vi "GenerateAnalogWaveformPiezoTraj - Copy.vi"(8 "error in (no error)":errorcluster, 11 "SetupInfo_IN":T1={"ConfigParameters_Analog"={"JAI camera fps"=240.0, "Bi-Lateral Galvo xy scan range (V)"=0.7, "Bi-Lateral Galvo xy scan frequency (Hz)"=500, "AOM Blind percent (%)"=0.1, "AOM start blind percent (%) "=70.0, "ROI threshold"=1.0, "AO Sampling rate"=1000000.0}, "ConfigParameters_Digital"={"Steps per volume"=25.0, "Time per volume (s)"=0.4, "OG start layer"=15.0, "Objective Lin Rising Vel (micron/ms）"=1.0, "Image depth (micron)"=200.0, "OG latency (s)"=10.0, "OG repitation"=3.0, "OG end layer"=17.0, "Shock1 duration (s)"=0.001, "Shock2 duration (s)"=0.001, "Shock3 duration (s)"=0.01, "Shock4 duration (s)"=0.01, "Shock5 duration (s)"=0.1, "Shock duration_New"=[]}, "ConfigParameters_Other1"={"Frontal Galvo xy scan range (V)"=0.14, "Frontal Galvo xy scan frequency (Hz)"=500, "PFI 0 digital clock frequency"=500000.0, "Window size for layer index"=0.5, "sCMOS fps"=95.0}, "ConfigParameters_Others2"={"#Trials baseline"=6, "#Trials test"=6, "Time before acq. (s)"=360.0, "Time before test (s)"=600.0, "#Blocks acquisition"=5, "Inter-trial interval baseline (s)"=60.0, "#Trials per acquition block"=6, "Inter-block interval acquisition (s)"=360.0, "Inter-trial interval acquisition (s)"=20.0, "Flash latency (s)"=10.0, "Flash duration (s)"=3.2, "Response duration (s)"=10.0, "MaxTimeEventDetection (s)"=6, "StimType"=enum."Flash", "#MaxEvents"=6}, "ProcessParametersOut"={"stand Z vol Acquisition time (s)"=0.2631578947368421, "stand Z vol Backward time (s)"=0.13684210526315793, "Objective scan volt"=5.0, "Bi-lateral Galvo Z scan volt"=0.45, "Frontal Galvo Z scan volt"=0.37, "Objective step length (micron)"=8.0, "OG Z volet Linear Dec time (s)"=0.024, "OG Z vol Stim. steps time (s)"=0.031578947368421054, "OG Z vol Linear Acc time (s)"=0.112, "#Vol. of flash"=8, "#Vol. of shock"=1, "#Vol. bef flash"=25, "#Vol. aft flash"=17, "OG Z vol Linear Dec time (s)"=0.112, "OG Z vol time (s)"=0.39073684210526316, "Stack duration"=[0.001, 0.001, 0.01, 0.01, 0.1], "AOM stand. value size"=400000, "Plane indexing length"=0, "#Vol. blank"=0, "#Vol. blank before acq"=0, "#Vol. blank before test"=0, " #Inter-block interval acquisition (Ed-St Vol)"=0}, "WaveformParameters"={"stand Z vol Acquisition samp info"={"Fs"=1000000.0, "#s"=263158.0}, "stand Z vol Backward samp info"={"Fs"=1000000.0, "#s"=136842.0}, "OG Z vol Linear Acc samp info"={"Fs"=1000000.0, "#s"=112000.0}, "OG Z vol Stim. steps samp info"={"Fs"=1000000.0, "#s"=31579.0}, "OG Z volet Linear Dec samp info"={"Fs"=1000000.0, "#s"=24000.0}, "OG Z vol Linear Dec samp info"={"Fs"=1000000.0, "#s"=112000.0}, "OG Z vol samp info"={"Fs"=1000000.0, "#s"=390737.0}, "stand Z vol backforth samp info"={"Fs"=1000000.0, "#s"=400000.0}}, "AnalogWaveform"={"Bi-lateral Galvo Z stand waveform"={"t0"=timestamp(0 s since 1904-01-01), "dt"=1.0, "Y"=[]}, "Frontal Galvo Z stand waveform"={"t0"=timestamp(0 s since 1904-01-01), "dt"=1.0, "Y"=[]}, "Bi-lateral Galvo XY stand waveform"={"t0"=timestamp(0 s since 1904-01-01), "dt"=1.0, "Y"=[]}, "Frontal Galvo XY stand waveform"={"t0"=timestamp(0 s since 1904-01-01), "dt"=1.0, "Y"=[]}, "sCMOS stand waveform"={"t0"=timestamp(0 s since 1904-01-01), "dt"=1.0, "Y"=[]}, "Detection objective stand waveform"={"t0"=timestamp(0 s since 1904-01-01), "dt"=1.0, "Y"=[]}, "AOM stand waveform"={"t0"=timestamp(0 s since 1904-01-01), "dt"=1.0, "Y"=[]}, "PFI 0 clock stand waveform"={"t0"=timestamp(0 s since 1904-01-01), "dt"=1.0, "Y"=[]}, "Bi-lateral Galvo Z OG waveform"={"t0"=timestamp(0 s since 1904-01-01), "dt"=1.0, "Y"=[]}, "Bi-lateral Galvo XY OG waveform"={"t0"=timestamp(0 s since 1904-01-01), "dt"=1.0, "Y"=[]}, "Frontal Galvo Z OG waveform"={"t0"=timestamp(0 s since 1904-01-01), "dt"=1.0, "Y"=[]}, "Frontal Galvo XY OG waveform"={"t0"=timestamp(0 s since 1904-01-01), "dt"=1.0, "Y"=[]}, "sCMOS OG waveform"={"t0"=timestamp(0 s since 1904-01-01), "dt"=1.0, "Y"=[]}, "Detection objective OG waveform"={"t0"=timestamp(0 s since 1904-01-01), "dt"=1.0, "Y"=[]}, "AOM OG waveform"={"t0"=timestamp(0 s since 1904-01-01), "dt"=1.0, "Y"=[]}, "PFI 0 clock OG wavee"={"t0"=timestamp(0 s since 1904-01-01), "dt"=1.0, "Y"=[]}, "sCMOS blank waveform"={"t0"=timestamp(0 s since 1904-01-01), "dt"=1.0, "Y"=[]}, "All analog OG wave"=[], "All analog stand wave"=[], "All analog blank wave"=[], "BufferWaveform_Analog"=[], "Bi-lateral Galvo Z XY"={"t0"=timestamp(0 s since 1904-01-01), "dt"=1.0, "Y"=[]}, "Frontal Galvo Z XY"={"t0"=timestamp(0 s since 1904-01-01), "dt"=1.0, "Y"=[]}, "sCMOS Trigger XY"={"t0"=timestamp(0 s since 1904-01-01), "dt"=1.0, "Y"=[]}, "Detection objective XY"={"t0"=timestamp(0 s since 1904-01-01), "dt"=1.0, "Y"=[]}, "AOM XY"={"t0"=timestamp(0 s since 1904-01-01), "dt"=1.0, "Y"=[]}, "Analog_XY"=[]}, "DigitalWaveform"={"AllDigitalStandWave"=[], "AllDigialEvokedWave"=[], "AllDigialOGWave"=[], "AllDigitalPairWave_1"=[], "AllDigitalPairWave_2"=[], "AllDigitalPairWave_3"=[], "AllDigitalPairWave_4"=[], "AllDigitalPairWave_5"=[], "Plane Indexing"={"t0"=timestamp(0 s since 1904-01-01), "dt"=0.0, "Y"={"transitions"=[], "data"=[]}, "error"={"status"=FALSE, "code"=37421928, "source"=""}}, "Plane indexing P0.5 OG"={"t0"=timestamp(0 s since 1904-01-01), "dt"=0.0, "Y"={"transitions"=[], "data"=[]}, "error"={"status"=FALSE, "code"=37421928, "source"=""}}, "AllDigitalPairWaves"=[], "BufferWaveform_Digital"=[], "AllDigitalBlankWave"=[], "Digial_XY"=[], "Digital_XY_flash"=[]}, "PhysicalResource"={"PhysicalChannels_AI"="", "PhysicalChannels_AO"="", "PhysicalChannels_DO"="", "Task_AnalogOutput"="", "Task_DigitalOutput"="", "Task_AnalogInput"=""}, "ControlsRef"={"Mode_1"=refnum, "EventDetectionMode"=refnum, "Mode_2A"=refnum, "StimulationMode"=refnum, "Mode_2B"=refnum, "ErrorMeg"=refnum}} {"ConfigParameters_Other1"."Frontal Galvo xy scan frequency (Hz)" min=500 max=500; "ConfigParameters_Other1"."Frontal Galvo xy scan range (V)" min=0.0 max=1.5; "ConfigParameters_Analog"."AOM start blind percent (%)" min=10.0 max=90.0; "ConfigParameters_Analog"."AOM Blind percent (%)" min=0.1 max=100.0; "ConfigParameters_Analog"."Bi-Lateral Galvo xy scan frequency (Hz)" min=500 max=500; "ConfigParameters_Analog"."Bi-Lateral Galvo xy scan range (V)" min=0.0 max=1.5}) -> (0 "error out":errorcluster, 3 "SetupInfo_OUT":T1={"ConfigParameters_Analog"={"JAI camera fps"=240.0, "Bi-Lateral Galvo xy scan range (V)"=0.7, "Bi-Lateral Galvo xy scan frequency (Hz)"=500, "AOM Blind percent (%)"=0.1, "AOM start blind percent (%) "=70.0, "ROI threshold"=1.0, "AO Sampling rate"=1000000.0}, "ConfigParameters_Digital"={"Steps per volume"=25.0, "Time per volume (s)"=0.4, "OG start layer"=15.0, "Objective Lin Rising Vel (micron/ms）"=1.0, "Image depth (micron)"=200.0, "OG latency (s)"=10.0, "OG repitation"=3.0, "OG end layer"=17.0, "Shock1 duration (s)"=0.001, "Shock2 duration (s)"=0.001, "Shock3 duration (s)"=0.01, "Shock4 duration (s)"=0.01, "Shock5 duration (s)"=0.1, "Shock duration_New"=[]}, "ConfigParameters_Other1"={"Frontal Galvo xy scan range (V)"=0.14, "Frontal Galvo xy scan frequency (Hz)"=500, "PFI 0 digital clock frequency"=500000.0, "Window size for layer index"=0.5, "sCMOS fps"=95.0}, "ConfigParameters_Others2"={"#Trials baseline"=6, "#Trials test"=6, "Time before acq. (s)"=360.0, "Time before test (s)"=600.0, "#Blocks acquisition"=5, "Inter-trial interval baseline (s)"=60.0, "#Trials per acquition block"=6, "Inter-block interval acquisition (s)"=360.0, "Inter-trial interval acquisition (s)"=20.0, "Flash latency (s)"=10.0, "Flash duration (s)"=3.2, "Response duration (s)"=10.0, "MaxTimeEventDetection (s)"=6, "StimType"=enum."Flash", "#MaxEvents"=6}, "ProcessParametersOut"={"stand Z vol Acquisition time (s)"=0.2631578947368421, "stand Z vol Backward time (s)"=0.13684210526315793, "Objective scan volt"=5.0, "Bi-lateral Galvo Z scan volt"=0.1800000180000018, "Frontal Galvo Z scan volt"=0.14940000509752818, "Objective step length (micron)"=8.0, "OG Z volet Linear Dec time (s)"=0.024, "OG Z vol Stim. steps time (s)"=0.031578947368421054, "OG Z vol Linear Acc time (s)"=0.112, "#Vol. of flash"=8, "#Vol. of shock"=1, "#Vol. bef flash"=25, "#Vol. aft flash"=17, "OG Z vol Linear Dec time (s)"=0.112, "OG Z vol time (s)"=0.39073684210526316, "Stack duration"=[0.001, 0.001, 0.01, 0.01, 0.1], "AOM stand. value size"=400000, "Plane indexing length"=0, "#Vol. blank"=0, "#Vol. blank before acq"=0, "#Vol. blank before test"=0, " #Inter-block interval acquisition (Ed-St Vol)"=0}, "WaveformParameters"={"stand Z vol Acquisition samp info"={"Fs"=1000000.0, "#s"=263158.0}, "stand Z vol Backward samp info"={"Fs"=1000000.0, "#s"=136842.0}, "OG Z vol Linear Acc samp info"={"Fs"=1000000.0, "#s"=112000.0}, "OG Z vol Stim. steps samp info"={"Fs"=1000000.0, "#s"=31579.0}, "OG Z volet Linear Dec samp info"={"Fs"=1000000.0, "#s"=24000.0}, "OG Z vol Linear Dec samp info"={"Fs"=1000000.0, "#s"=112000.0}, "OG Z vol samp info"={"Fs"=1000000.0, "#s"=390737.0}, "stand Z vol backforth samp info"={"Fs"=1000000.0, "#s"=400000.0}}, "AnalogWaveform"={"Bi-lateral Galvo Z stand waveform"={"t0"=timestamp(0 s since 1904-01-01), "dt"=1.0, "Y"=[]}, "Frontal Galvo Z stand waveform"={"t0"=timestamp(0 s since 1904-01-01), "dt"=1.0, "Y"=[]}, "Bi-lateral Galvo XY stand waveform"={"t0"=timestamp(0 s since 1904-01-01), "dt"=1.0, "Y"=[]}, "Frontal Galvo XY stand waveform"={"t0"=timestamp(0 s since 1904-01-01), "dt"=1.0, "Y"=[]}, "sCMOS stand waveform"={"t0"=timestamp(0 s since 1904-01-01), "dt"=1.0, "Y"=[]}, "Detection objective stand waveform"={"t0"=timestamp(0 s since 1904-01-01), "dt"=1.0, "Y"=[]}, "AOM stand waveform"={"t0"=timestamp(0 s since 1904-01-01), "dt"=1.0, "Y"=[]}, "PFI 0 clock stand waveform"={"t0"=timestamp(0 s since 1904-01-01), "dt"=1.0, "Y"=[]}, "Bi-lateral Galvo Z OG waveform"={"t0"=timestamp(0 s since 1904-01-01), "dt"=1.0, "Y"=[]}, "Bi-lateral Galvo XY OG waveform"={"t0"=timestamp(0 s since 1904-01-01), "dt"=1.0, "Y"=[]}, "Frontal Galvo Z OG waveform"={"t0"=timestamp(0 s since 1904-01-01), "dt"=1.0, "Y"=[]}, "Frontal Galvo XY OG waveform"={"t0"=timestamp(0 s since 1904-01-01), "dt"=1.0, "Y"=[]}, "sCMOS OG waveform"={"t0"=timestamp(0 s since 1904-01-01), "dt"=1.0, "Y"=[]}, "Detection objective OG waveform"={"t0"=timestamp(0 s since 1904-01-01), "dt"=1.0, "Y"=[]}, "AOM OG waveform"={"t0"=timestamp(0 s since 1904-01-01), "dt"=1.0, "Y"=[]}, "PFI 0 clock OG wavee"={"t0"=timestamp(0 s since 1904-01-01), "dt"=1.0, "Y"=[]}, "sCMOS blank waveform"={"t0"=timestamp(0 s since 1904-01-01), "dt"=1.0, "Y"=[]}, "All analog OG wave"=[], "All analog stand wave"=[], "All analog blank wave"=[], "BufferWaveform_Analog"=[], "Bi-lateral Galvo Z XY"={"t0"=timestamp(0 s since 1904-01-01), "dt"=1.0, "Y"=[]}, "Frontal Galvo Z XY"={"t0"=timestamp(0 s since 1904-01-01), "dt"=1.0, "Y"=[]}, "sCMOS Trigger XY"={"t0"=timestamp(0 s since 1904-01-01), "dt"=1.0, "Y"=[]}, "Detection objective XY"={"t0"=timestamp(0 s since 1904-01-01), "dt"=1.0, "Y"=[]}, "AOM XY"={"t0"=timestamp(0 s since 1904-01-01), "dt"=1.0, "Y"=[]}, "Analog_XY"=[]}, "DigitalWaveform"={"AllDigitalStandWave"=[], "AllDigialEvokedWave"=[], "AllDigialOGWave"=[], "AllDigitalPairWave_1"=[], "AllDigitalPairWave_2"=[], "AllDigitalPairWave_3"=[], "AllDigitalPairWave_4"=[], "AllDigitalPairWave_5"=[], "Plane Indexing"={"t0"=timestamp(0 s since 1904-01-01), "dt"=0.0, "Y"={"transitions"=[], "data"=[]}, "error"={"status"=FALSE, "code"=37421928, "source"=""}}, "Plane indexing P0.5 OG"={"t0"=timestamp(0 s since 1904-01-01), "dt"=0.0, "Y"={"transitions"=[], "data"=[]}, "error"={"status"=FALSE, "code"=37421928, "source"=""}}, "AllDigitalPairWaves"=[], "BufferWaveform_Digital"=[], "AllDigitalBlankWave"=[], "Digial_XY"=[], "Digital_XY_flash"=[]}, "PhysicalResource"={"PhysicalChannels_AI"="", "PhysicalChannels_AO"="", "PhysicalChannels_DO"="", "Task_AnalogOutput"="", "Task_DigitalOutput"="", "Task_AnalogInput"=""}, "ControlsRef"={"Mode_1"=refnum, "EventDetectionMode"=refnum, "Mode_2A"=refnum, "StimulationMode"=refnum, "Mode_2B"=refnum, "ErrorMeg"=refnum}} {"ConfigParameters_Other1"."Frontal Galvo xy scan frequency (Hz)" min=500 max=500; "ConfigParameters_Other1"."Frontal Galvo xy scan range (V)" min=0.0 max=1.5; "ConfigParameters_Analog"."AOM start blind percent (%)" min=10.0 max=90.0; "ConfigParameters_Analog"."AOM Blind percent (%)" min=0.1 max=100.0; "ConfigParameters_Analog"."Bi-Lateral Galvo xy scan frequency (Hz)" min=500 max=500; "ConfigParameters_Analog"."Bi-Lateral Galvo xy scan range (V)" min=0.0 max=1.5})   [LabVIEW 2018]
uses:
  SetupInfo.ctl
  ConfigParameters_Analog.ctl
  ConfigParameters_Digital.ctl
  ConfigParameters_Others1.ctl
  ConfigParameters_Others2.ctl
  ProcessParametersOut.ctl
  WaveformParameters.ctl
  AnalogWaveform.ctl
  DigitalWaveform.ctl
  PhysicalResource.ctl
  ControlsRef.ctl
  <vilib>/Waveform/WDTOps.llb/WDT Append Waveforms DBL.vi
  <vilib>/measure/NI_MABase.lvlib
panel:
  in  "FileSamplingRate":dbl=1000.0
  in  "PiezoTrajectoryPath":path=path "D:/APP/LightSheetController_Ver8 obl/VISource/Waveform/Piezo_feedback_20201106.txt"
  out "AOM stand. value size":i32=400000
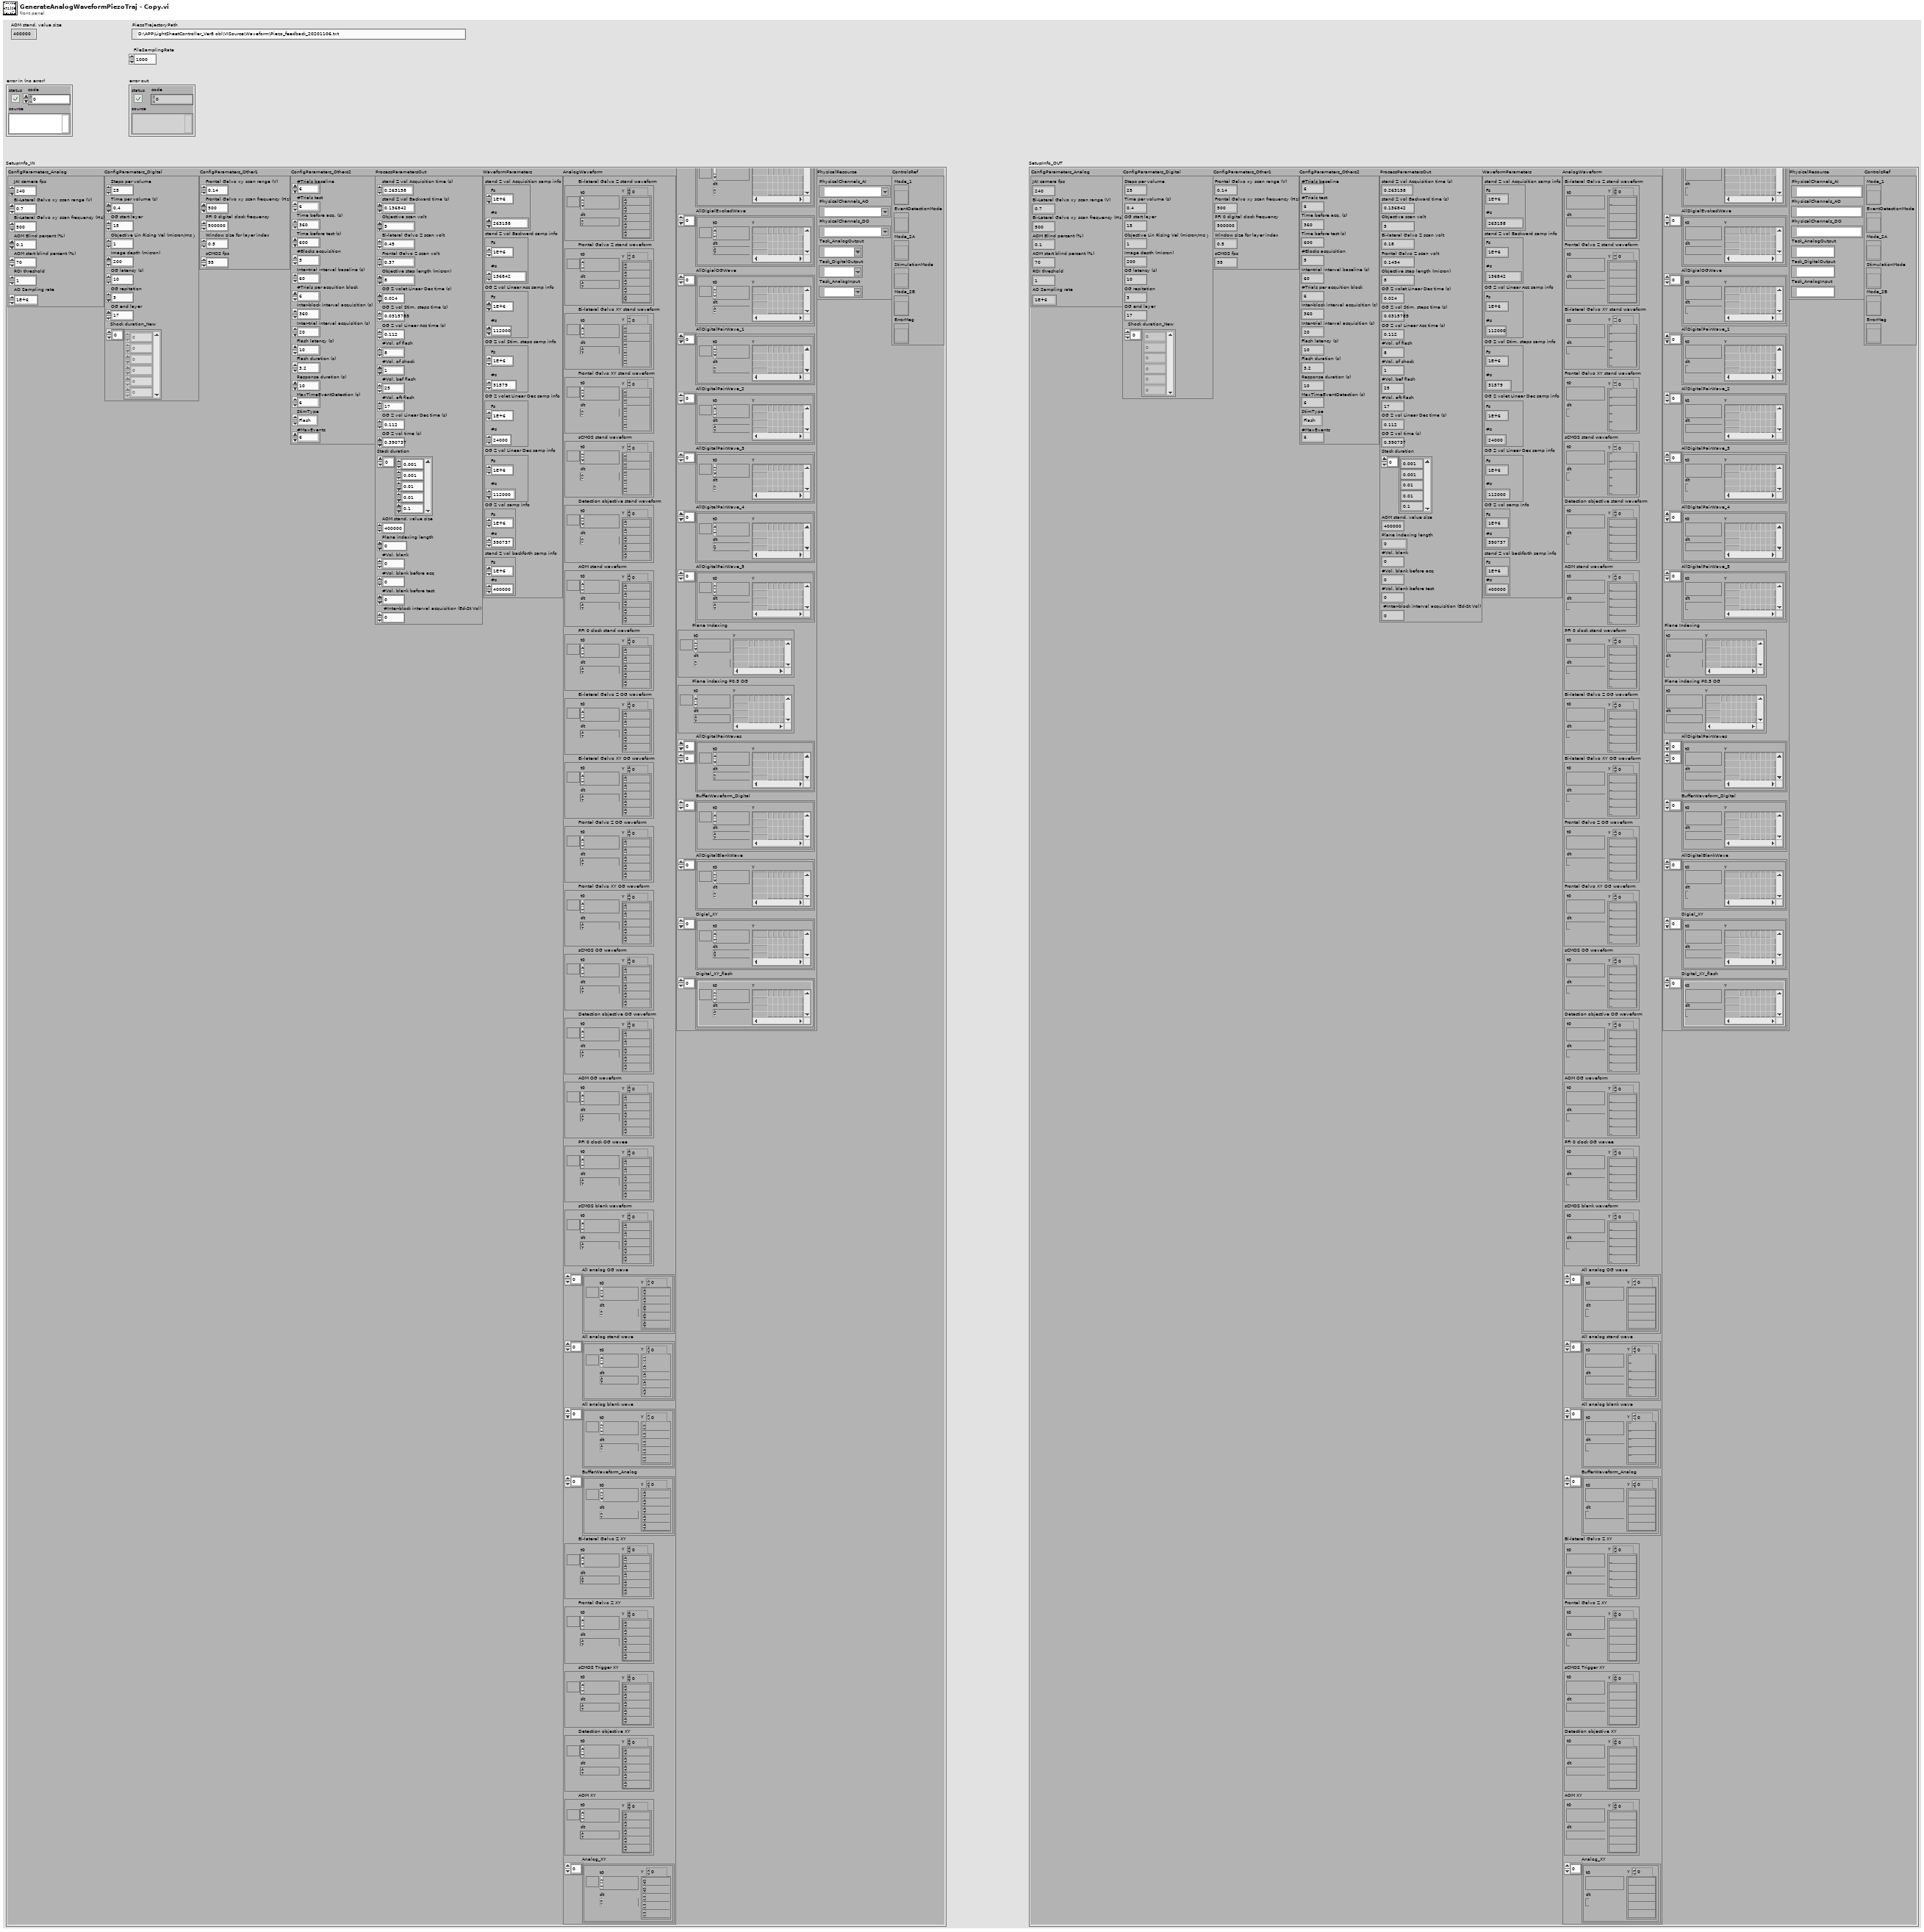
[diagram p1: front panel]
types:
  T1 = typedef "SetupInfo.ctl" = cluster{"ConfigParameters_Analog":T2, "ConfigParameters_Digital":T3, "ConfigParameters_Other1":T4, "ConfigParameters_Others2":T5, "ProcessParametersOut":T6, "WaveformParameters":T7, "AnalogWaveform":T8, "DigitalWaveform":T9, "PhysicalResource":T10, "ControlsRef":T11}
  T2 = typedef "ConfigParameters_Analog.ctl" = cluster{"JAI camera fps":dbl, "Bi-Lateral Galvo xy scan range (V)":dbl, "Bi-Lateral Galvo xy scan frequency (Hz)":i16, "AOM Blind percent (%)":dbl, "AOM start blind percent (%) ":dbl, "ROI threshold":dbl, "AO Sampling rate":dbl}
  T3 = typedef "ConfigParameters_Digital.ctl" = cluster{"Steps per volume":dbl, "Time per volume (s)":dbl, "OG start layer":dbl, "Objective Lin Rising Vel (micron/ms）":dbl, "Image depth (micron)":dbl, "OG latency (s)":dbl, "OG repitation":dbl, "OG end layer":dbl, "Shock1 duration (s)":dbl, "Shock2 duration (s)":dbl, "Shock3 duration (s)":dbl, "Shock4 duration (s)":dbl, "Shock5 duration (s)":dbl, "Shock duration_New":dbl[]}
  T4 = typedef "ConfigParameters_Others1.ctl" = cluster{"Frontal Galvo xy scan range (V)":dbl, "Frontal Galvo xy scan frequency (Hz)":i16, "PFI 0 digital clock frequency":dbl, "Window size for layer index":dbl, "sCMOS fps":dbl}
  T5 = typedef "ConfigParameters_Others2.ctl" = cluster{"#Trials baseline":i32, "#Trials test":i32, "Time before acq. (s)":dbl, "Time before test (s)":dbl, "#Blocks acquisition":i32, "Inter-trial interval baseline (s)":dbl, "#Trials per acquition block":i32, "Inter-block interval acquisition (s)":dbl, "Inter-trial interval acquisition (s)":dbl, "Flash latency (s)":dbl, "Flash duration (s)":dbl, "Response duration (s)":dbl, "MaxTimeEventDetection (s)":i32, "StimType":enum16{"Flash", "OG"}, "#MaxEvents":i32}
  T6 = typedef "ProcessParametersOut.ctl" = cluster{"stand Z vol Acquisition time (s)":dbl, "stand Z vol Backward time (s)":dbl, "Objective scan volt":dbl, "Bi-lateral Galvo Z scan volt":dbl, "Frontal Galvo Z scan volt":dbl, "Objective step length (micron)":dbl, "OG Z volet Linear Dec time (s)":dbl, "OG Z vol Stim. steps time (s)":dbl, "OG Z vol Linear Acc time (s)":dbl, "#Vol. of flash":i32, "#Vol. of shock":i32, "#Vol. bef flash":i32, "#Vol. aft flash":i32, "OG Z vol Linear Dec time (s)":dbl, "OG Z vol time (s)":dbl, "Stack duration":dbl[], "AOM stand. value size":i32, "Plane indexing length":i32, "#Vol. blank":i32, "#Vol. blank before acq":i32, "#Vol. blank before test":i32, " #Inter-block interval acquisition (Ed-St Vol)":i32}
  T7 = typedef "WaveformParameters.ctl" = cluster{"stand Z vol Acquisition samp info":cluster{"Fs":dbl, "#s":dbl}, "stand Z vol Backward samp info":cluster{"Fs":dbl, "#s":dbl}, "OG Z vol Linear Acc samp info":cluster{"Fs":dbl, "#s":dbl}, "OG Z vol Stim. steps samp info":cluster{"Fs":dbl, "#s":dbl}, "OG Z volet Linear Dec samp info":cluster{"Fs":dbl, "#s":dbl}, "OG Z vol Linear Dec samp info":cluster{"Fs":dbl, "#s":dbl}, "OG Z vol samp info":cluster{"Fs":dbl, "#s":dbl}, "stand Z vol backforth samp info":cluster{"Fs":dbl, "#s":dbl}}
  T8 = typedef "AnalogWaveform.ctl" = cluster{"Bi-lateral Galvo Z stand waveform":waveform(dbl), "Frontal Galvo Z stand waveform":waveform(dbl), "Bi-lateral Galvo XY stand waveform":waveform(dbl), "Frontal Galvo XY stand waveform":waveform(dbl), "sCMOS stand waveform":waveform(dbl), "Detection objective stand waveform":waveform(dbl), "AOM stand waveform":waveform(dbl), "PFI 0 clock stand waveform":waveform(dbl), "Bi-lateral Galvo Z OG waveform":waveform(dbl), "Bi-lateral Galvo XY OG waveform":waveform(dbl), "Frontal Galvo Z OG waveform":waveform(dbl), "Frontal Galvo XY OG waveform":waveform(dbl), "sCMOS OG waveform":waveform(dbl), "Detection objective OG waveform":waveform(dbl), "AOM OG waveform":waveform(dbl), "PFI 0 clock OG wavee":waveform(dbl), "sCMOS blank waveform":waveform(dbl), "All analog OG wave":waveform(dbl)[], "All analog stand wave":waveform(dbl)[], "All analog blank wave":waveform(dbl)[], "BufferWaveform_Analog":waveform(dbl)[], "Bi-lateral Galvo Z XY":waveform(dbl), "Frontal Galvo Z XY":waveform(dbl), "sCMOS Trigger XY":waveform(dbl), "Detection objective XY":waveform(dbl), "AOM XY":waveform(dbl), "Analog_XY":waveform(dbl)[]}
  T9 = typedef "DigitalWaveform.ctl" = cluster{"AllDigitalStandWave":digitalwaveform[], "AllDigialEvokedWave":digitalwaveform[], "AllDigialOGWave":digitalwaveform[], "AllDigitalPairWave_1":digitalwaveform[], "AllDigitalPairWave_2":digitalwaveform[], "AllDigitalPairWave_3":digitalwaveform[], "AllDigitalPairWave_4":digitalwaveform[], "AllDigitalPairWave_5":digitalwaveform[], "Plane Indexing":digitalwaveform, "Plane indexing P0.5 OG":digitalwaveform, "AllDigitalPairWaves":digitalwaveform[][], "BufferWaveform_Digital":digitalwaveform[], "AllDigitalBlankWave":digitalwaveform[], "Digial_XY":digitalwaveform[], "Digital_XY_flash":digitalwaveform[]}
  T10 = typedef "PhysicalResource.ctl" = cluster{"PhysicalChannels_AI":tag, "PhysicalChannels_AO":tag, "PhysicalChannels_DO":tag, "Task_AnalogOutput":refnum<k21>, "Task_DigitalOutput":refnum<k21>, "Task_AnalogInput":refnum<k21>}
  T11 = typedef "ControlsRef.ctl" = cluster{"Mode_1":refnum<vi>, "EventDetectionMode":refnum<vi>, "Mode_2A":refnum<vi>, "StimulationMode":refnum<vi>, "Mode_2B":refnum<vi>, "ErrorMeg":refnum<vi>}
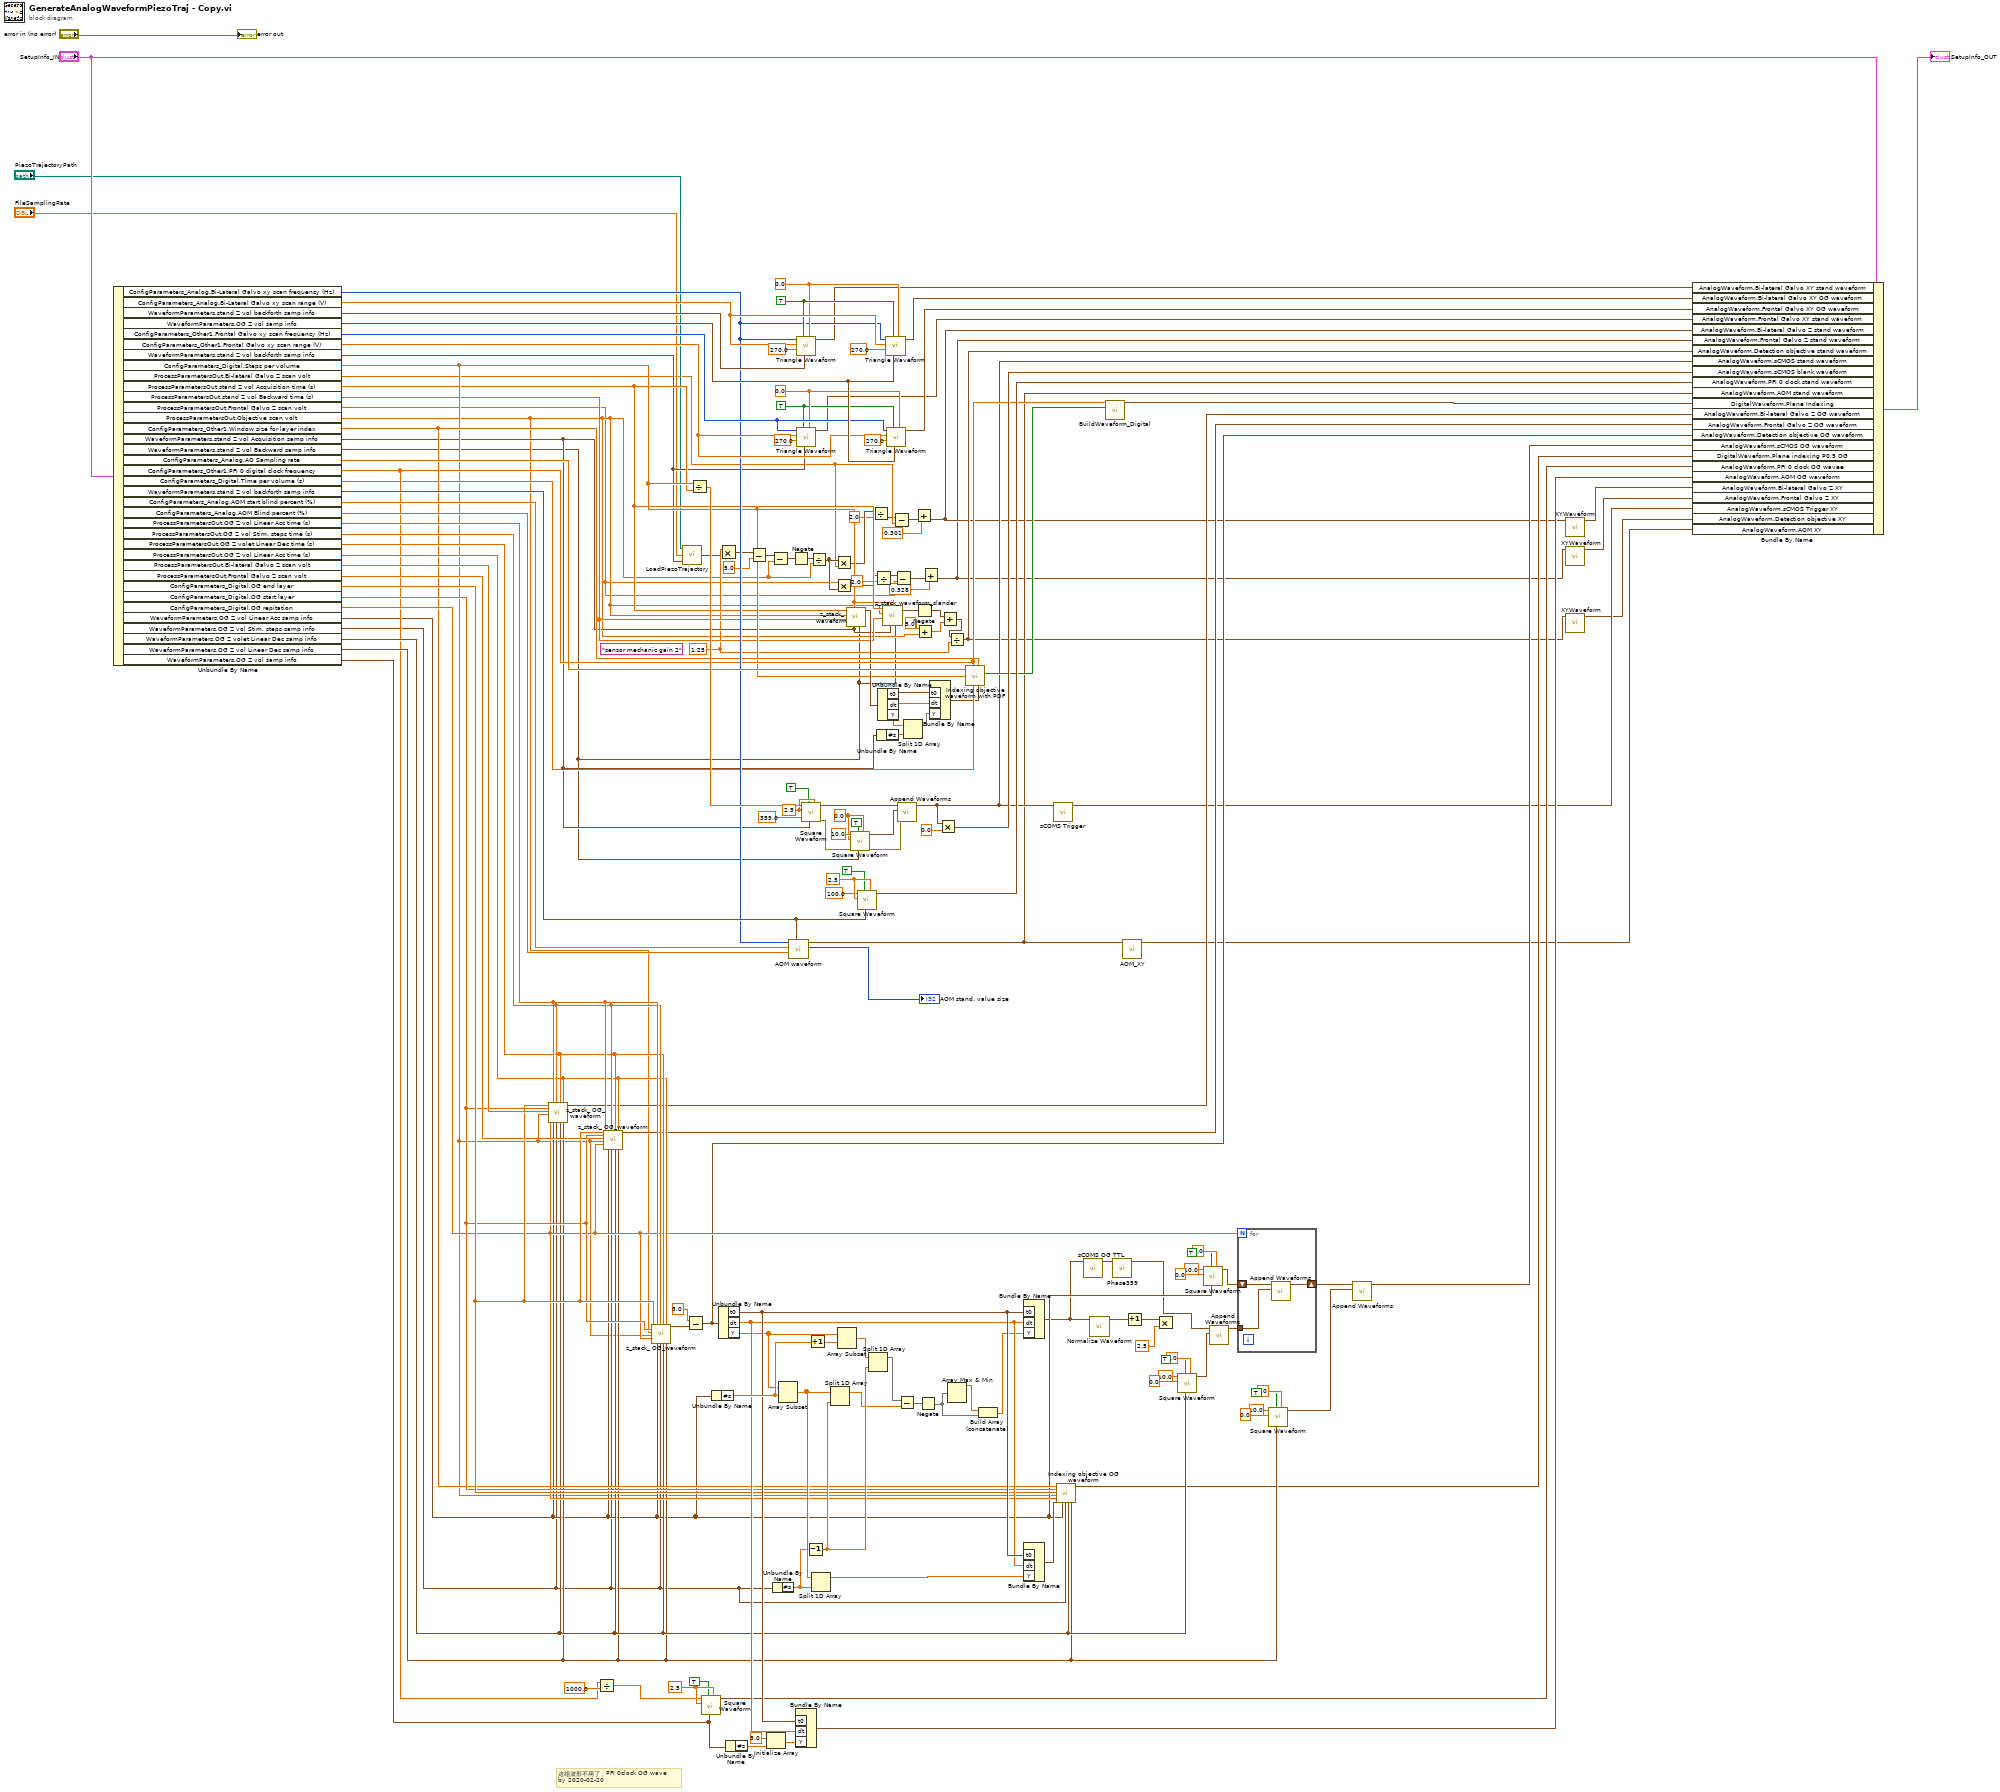
[diagram p0: block diagram]
diagram:
  (unwired) "sensor mechanic gain 2"
  w26 = 1.25
  w99 = 2.5
  w144 = 2.5 ("offset")
  w151 = 0.0 ("offset")
  w155 = 2.5 ("amplitude")
  w130 = TRUE ("reset signal")
  w138 = TRUE ("reset signal")
  w137 = 0.0 ("offset")
  w131 = 0.0 ("offset")
  # "这组波形不用了，PFI 0clock OG wave\nby 2020-02-20"
  n1 = Unbundle By Name("SetupInfo_IN") -> ("ConfigParameters_Analog.Bi-Lateral Galvo xy scan frequency (Hz)"=w126:i16, "ConfigParameters_Analog.Bi-Lateral Galvo xy scan range (V)"=w140:dbl, "WaveformParameters.stand Z vol backforth samp info"=w139:cluster{"Fs":dbl, "#s":dbl}, "WaveformParameters.OG Z vol samp info"=w135:cluster{"Fs":dbl, "#s":dbl}, "ConfigParameters_Other1.Frontal Galvo xy scan frequency (Hz)"=w134:i16, "ConfigParameters_Other1.Frontal Galvo xy scan range (V)"=w133:dbl, "WaveformParameters.stand Z vol backforth samp info"=w28:cluster{"Fs":dbl, "#s":dbl}, "ConfigParameters_Digital.Steps per volume"=w34:dbl, "ProcessParametersOut.Bi-lateral Galvo Z scan volt"=w10:dbl, "ProcessParametersOut.stand Z vol Acquisition time (s)"=w33:dbl, "ProcessParametersOut.stand Z vol Backward time (s)"=w32:dbl, "ProcessParametersOut.Frontal Galvo Z scan volt"=w11:dbl, "ProcessParametersOut.Objective scan volt"=w19:dbl, "ConfigParameters_Other1.Window size for layer index"=w83:dbl, "WaveformParameters.stand Z vol Acquisition samp info"=w31:cluster{"Fs":dbl, "#s":dbl}, "WaveformParameters.stand Z vol Backward samp info"=w17:cluster{"Fs":dbl, "#s":dbl}, "ConfigParameters_Analog.AO Sampling rate"=w128:dbl, "ConfigParameters_Other1.PFI 0 digital clock frequency"=w67:dbl, "ConfigParameters_Digital.Time per volume (s)"=w66:dbl, "WaveformParameters.stand Z vol backforth samp info"=w127:cluster{"Fs":dbl, "#s":dbl}, "ConfigParameters_Analog.AOM start blind percent (%)"=w125:dbl, "ConfigParameters_Analog.AOM Blind percent (%)"=w124:dbl, "ProcessParametersOut.OG Z vol Linear Acc time (s)"=w92:dbl, "ProcessParametersOut.OG Z vol Stim. steps time (s)"=w91:dbl, "ProcessParametersOut.OG Z volet Linear Dec time (s)"=w90:dbl, "ProcessParametersOut.OG Z vol Linear Acc time (s)"=w89:dbl, "ProcessParametersOut.Bi-lateral Galvo Z scan volt"=w88:dbl, "ProcessParametersOut.Frontal Galvo Z scan volt"=w87:dbl, "ConfigParameters_Digital.OG end layer"=w86:dbl, "ConfigParameters_Digital.OG start layer"=w85:dbl, "ConfigParameters_Digital.OG repitation"=w84:dbl, "WaveformParameters.OG Z vol Linear Acc samp info"=w49:cluster{"Fs":dbl, "#s":dbl}, "WaveformParameters.OG Z vol Stim. steps samp info"=w48:cluster{"Fs":dbl, "#s":dbl}, "WaveformParameters.OG Z volet Linear Dec samp info"=w82:cluster{"Fs":dbl, "#s":dbl}, "WaveformParameters.OG Z vol Linear Dec samp info"=w81:cluster{"Fs":dbl, "#s":dbl}, "WaveformParameters.OG Z vol samp info"=w80:cluster{"Fs":dbl, "#s":dbl})
  n2 = call "z_stack_ OG_waveform.vi"("OG end layer"=w86, "OG start layer"=w85, "SPECIFIC scan volt"=w88, "Steps per volume"=w34, "OG repitation"=w84, "Objective线性加速时间"=w92, "OG Z stack 线性加速 采样信息"=w49, "Objective 刺激steps 时间（s）"=w91, "OG Z stack 刺激steps 采样信息"=w48, "Objective volet 线性减速 时间（s）"=w90, "OG Z volet 线性减速 采样信息"=w82, "Objective线性减速时间"=w89, "OG Z stack 线性减速 采样信息"=w81) -> ("waveform out"=w70:waveform(dbl))  [unwired: 2 in, 4 out]
  n3 = Divide(x=w67, y=1000.0) -> (x/y=w73:dbl)
  n4 = call "z_stack_ OG_waveform.vi"("OG end layer"=w86, "OG start layer"=w85, "SPECIFIC scan volt"=w87, "Steps per volume"=w34, "OG repitation"=w84, "Objective线性加速时间"=w92, "OG Z stack 线性加速 采样信息"=w49, "Objective 刺激steps 时间（s）"=w91, "OG Z stack 刺激steps 采样信息"=w48, "Objective volet 线性减速 时间（s）"=w90, "OG Z volet 线性减速 采样信息"=w82, "Objective线性减速时间"=w89, "OG Z stack 线性减速 采样信息"=w81) -> ("waveform out"=w69:waveform(dbl))  [unwired: 2 in, 4 out]
  n5 = call "z_stack_ OG_waveform.vi"("OG end layer"=w86, "OG start layer"=w85, "SPECIFIC scan volt"=w19, "Steps per volume"=w34, "OG repitation"=w84, "Objective线性加速时间"=w92, "OG Z stack 线性加速 采样信息"=w49, "Objective 刺激steps 时间（s）"=w91, "OG Z stack 刺激steps 采样信息"=w48, "Objective volet 线性减速 时间（s）"=w90, "OG Z volet 线性减速 采样信息"=w82, "Objective线性减速时间"=w89, "OG Z stack 线性减速 采样信息"=w81) -> ("waveform out"=w62:waveform(dbl))  [unwired: 2 in, 4 out]
  n6 = call "LoadPiezoTrajactory.vi"("Z backforth 采样信息"=w28, "File Sampling Rate"="FileSamplingRate", "Path"="PiezoTrajectoryPath") -> ("output waveform"=w14:waveform(dbl))
  n7 = Subtract(x=5.0, y=w62) -> (x-y=w57:waveform(dbl))
  n8 = Divide(x=w34, y=w33) -> (x/y=w156:dbl)
  n9 = call <vilib>:"Square Waveform.vi"("offset"=w99, "sampling info"=w80, "reset signal"=TRUE, "amplitude"=w99, "frequency"=w73) -> ("signal out"=w78:waveform(dbl))  [unwired: 5 in, 1 out]
  n10 = Unbundle By Name(w49) -> ("#s"=w100:dbl)
  n11 = Unbundle By Name(w57) -> ("t0"=w95:timestamp, "dt"=w94:dbl, "Y"=w60:dbl[])
  n12 = Multiply(x=w26, y=w14) -> (x*y=w25:waveform(dbl))
  n13 = Unbundle By Name(w80) -> ("#s"=w93:dbl)
  n14 = Subtract(x=w25, y=5.0) -> (x-y=w24:waveform(dbl))
  n15 = Initialize Array(5.0 ("element"), w93) -> (w96:dbl[])
  n16 = Subtract(x=w24, y=w19) -> (x-y=w21:waveform(dbl))
  n17 = Unbundle By Name(w48) -> ("#s"=w101:dbl)
  n18 = Array Subset(array=w60, index=w100) -> (w117:dbl[])  [unwired: 1 in]
  n19 = call "AOM waveform.vi"("z stack 往复采样信息"=w127, "AOM Blind percent (%)"=w124, "AOM start blind percent (%)"=w125, "Bi-Lateral Galvo xy scan frequency (Hz)"=w126) -> ("数值"=→"AOM stand. value size":i32, "Waveform"=w36:waveform(dbl))  [unwired: 6 in]
  n20 = Negate(x=w21) -> (-x=w20:waveform(dbl))
  n21 = Bundle By Name("t0"=w95, "dt"=w94, "Y"=w96) -> (w77:waveform(dbl))  [unwired: 1 in]
  n22 = call <vilib>:"Triangle Waveform.vi"("offset"=w137, "sampling info"=w139, "reset signal"=w138, "phase"=270.0, "amplitude"=w140, "frequency"=w126) -> ("signal out"=w75:waveform(dbl))  [unwired: 4 in, 1 out]
  n23 = call <vilib>:"Triangle Waveform.vi"("offset"=w131, "sampling info"=w28, "reset signal"=w130, "phase"=270.0, "amplitude"=w133, "frequency"=w134) -> ("signal out"=w129:waveform(dbl))  [unwired: 4 in, 1 out]
  n24 = call <vilib>:"Square Waveform.vi"("offset"=w155, "sampling info"=w31, "reset signal"=TRUE, "phase"=359.0, "amplitude"=w155, "frequency"=w156) -> ("error out"=w149:errorcluster, "signal out"=w147:waveform(dbl))  [unwired: 4 in]
  n25 = Decrement(x=w101) -> (x-1=w118:dbl)
  n26 = Increment(x=w100) -> (x+1=w119:dbl)
  n27 = Divide(x=w20, y=w19) -> (x/y=w18:waveform(dbl))
  n28 = Split 1D Array(array=w117, index=w101) -> (first subarray=w116:dbl[])  [unwired: 1 out]
  n29 = Split 1D Array(array=w117, index=w118) -> (first subarray=w53:dbl[])  [unwired: 1 out]
  n30 = Multiply(x=w18, y=w10) -> (x*y=w8:waveform(dbl))
  n31 = Multiply(x=w11, y=w18) -> (x*y=w13:waveform(dbl))
  n32 = Array Subset(array=w60, index=w119) -> (w59:dbl[])  [unwired: 1 in]
  n33 = call "z_stack_waveform.vi"("Z stack backward"=w17, "Z stack acquisition"=w31, "Steps per Volume"=w34, "Backward Time (s)"=w32, "SPECIFIC scan volt"=w19, "Aquisition Time (s)"=w33) -> ("WaveformOut"=w64:waveform(dbl))  [unwired: 5 in]
  n34 = call <vilib>:"Square Waveform.vi"("offset"=w151, "sampling info"=w17, "reset signal"=TRUE, "error in (no error)"=w149, "amplitude"=w151, "frequency"=10.0) -> ("error out"=w146:errorcluster, "signal out"=w148:waveform(dbl))  [unwired: 4 in]
  n35 = call <vilib>:"Square Waveform.vi"("offset"=w144, "sampling info"=w127, "reset signal"=TRUE, "amplitude"=w144, "frequency"=100.0 ("amplitude")) -> ("signal out"=w122:waveform(dbl))  [unwired: 5 in, 1 out]
  n36 = Split 1D Array(array=w59, index=w118) -> (first subarray=w54:dbl[])  [unwired: 1 out]
  n37 = Divide(x=w8, y=2.0) -> (x/y=w9:waveform(dbl))
  n38 = Divide(x=w13, y=2.0) -> (x/y=w6:waveform(dbl))
  n39 = Unbundle By Name(w31) -> ("#s"=w158:dbl)
  n40 = Unbundle By Name(w64) -> ("t0"=w161:timestamp, "dt"=w160:dbl, "Y"=w159:dbl[])
  n41 = call "z_stack_waveform_slander.vi"("Z stack backward"=w17, "Z stack acquisition"=w31, "Steps per Volume"=w34, "Backward Time (s)"=w32, "SPECIFIC scan volt"=w19, "Aquisition Time (s)"=w33) -> ("WaveformOut"=w35:waveform(dbl))  [unwired: 5 in]
  n42 = call <vilib>:"Triangle Waveform.vi"("offset"=w137, "sampling info"=w135, "reset signal"=w138, "phase"=270.0, "amplitude"=w140, "frequency"=w126) -> ("signal out"=w136:waveform(dbl))  [unwired: 4 in, 1 out]
  n43 = call <vilib>:"Triangle Waveform.vi"("offset"=w131, "sampling info"=w135, "reset signal"=w130, "phase"=270.0, "amplitude"=w133, "frequency"=w134) -> ("signal out"=w132:waveform(dbl))  [unwired: 4 in, 1 out]
  n44 = Subtract(x=w9, y=w10) -> (x-y=w12:waveform(dbl))
  n45 = Subtract(x=w6, y=w11) -> (x-y=w15:waveform(dbl))
  n46 = call-poly <vilib>:"Append Waveforms.vi"("error in (no error)"=w146, "waveform B"=w148, "waveform A"=w147) -> ("waveform out"=w40:waveform(dbl))  [unwired: 7 in, 1 out]
  n47 = Subtract(x=w54, y=w53) -> (x-y=w51:dbl[])
  n48 = Split 1D Array(array=w159, index=w158) -> (first subarray=w157:dbl[])  [unwired: 1 out]
  n49 = Add(x=0.301, y=w12) -> (x+y=w4:waveform(dbl))
  n50 = Negate(x=w35) -> (-x=w163:waveform(dbl))
  n51 = Add(x=5.0, y=w19) -> (x+y=w162:dbl)
  n52 = Negate(x=w51) -> (-x=w58:dbl[])
  n53 = Add(x=0.528, y=w15) -> (x+y=w3:waveform(dbl))
  n54 = Bundle By Name("t0"=w161, "dt"=w160, "Y"=w157) -> (w65:waveform(dbl))  [unwired: 1 in]
  n55 = Multiply(x=w40, y=0.0) -> (x*y=w123:waveform(dbl))
  n56 = Add(x=w163, y=w162) -> (x+y=w30:waveform(dbl))
  n57 = Divide(x=w30, y=w26) -> (x/y=w29:waveform(dbl))
  n58 = Array Max & Min(array=w58) -> (max value=w120:dbl)  [unwired: 3 out]
  n59 = call "Indexing objective waveform with PDF.vi"("AO sampling rate"=w128, "PFI0 digital clock frequency"=w67, "Steps per Volume"=w34, "Time per volume (s)"=w66, "Window size for layer index (ms)"=w83, "Steps Waveform"=w65) -> ("Plane Indexing data"=w72:bool[])  [unwired: 3 in, 1 out]
  n60 = Build Array (concatenate)(w120, w58) -> (w50:dbl[])
  n61 = Bundle By Name("t0"=w95, "dt"=w94, "Y"=w50) -> (w46:waveform(dbl))  [unwired: 1 in]
  n62 = Bundle By Name("t0"=w95, "dt"=w94, "Y"=w116) -> (w115:waveform(dbl))  [unwired: 1 in]
  n63 = call "sCOMS Trigger.vi"("In"=w40) -> ("Out"=w39:waveform(dbl))  [unwired: 10 in]
  n64 = call "Indexing objective OG waveform.vi"("Window size for layer index"=w83, "OG start layer"=w85, "OG end layer"=w86, "Steps per Volume"=w34, "OG repitation"=w84, "Waveform"=w115, "OG Z 线性加速 采样信息"=w49, "OG Z stack 刺激 steps 采样信息"=w48, "OG Z volet 线性减速 采样信息"=w82, "OG Z 线性减速 采样信息"=w81) -> ("Waveform_Digital"=w79:digitalwaveform)  [unwired: 9 in]
  n65 = call "sCOMS OG TTL.vi"("DataIn"=w46) -> ("Out"=w44:waveform(dbl))  [unwired: 10 in]
  n66 = call <vilib>:"Normalize Waveform.vi"("waveform in"=w46) -> ("normalized waveform"=w61:waveform(dbl))  [unwired: 7 in, 3 out]
  n67 = call "BuildWaveform_Digital.vi"("DigitalData"=w72, "SampleRate"=w67) -> ("DigitalWaveformOut"=w68:digitalwaveform)  [unwired: 9 in]
  n68 = call "Phase359.vi"("DataIn"=w44) -> ("DataOut"=w43:waveform(dbl))  [unwired: 10 in]
  n69 = call "AOM_XY.vi"("In"=w36) -> ("Out"=w37:waveform(dbl))  [unwired: 10 in]
  n70 = Increment(x=w61) -> (x+1=w63:waveform(dbl))
  n71 = Multiply(x=w63, y=2.5) -> ()  [unwired: 1 out]
  n72 = call <vilib>:"Square Waveform.vi"("offset"=0.0, "sampling info"=w82, "reset signal"=TRUE, "amplitude"=0.0, "frequency"=10.0) -> ("signal out"=w110:waveform(dbl))  [unwired: 5 in, 1 out]
  n73 = call <vilib>:"Square Waveform.vi"("offset"=0.0, "sampling info"=w49, "reset signal"=TRUE, "amplitude"=0.0, "frequency"=10.0) -> ("signal out"=w56:waveform(dbl))  [unwired: 5 in, 1 out]
  n74 = call-poly <vilib>:"Append Waveforms.vi"("waveform B"=w110, "waveform A"=w43) -> ("waveform out"=w55:waveform(dbl))  [unwired: 8 in, 1 out]
  n75 = for {
    N: w84 -> [_]
    tunnel: w55 -> [w172]
    shift-right: [w170] -> w47
    shift-left: w56 -> [w171]
    n76 = call-poly <vilib>:"Append Waveforms.vi"("waveform B"=w172, "waveform A"=w171) -> ("waveform out"=w170:waveform(dbl))  [unwired: 8 in, 1 out]
  }
  n77 = call <vilib>:"Square Waveform.vi"("offset"=0.0, "sampling info"=w81, "reset signal"=TRUE, "amplitude"=0.0, "frequency"=10.0) -> ("signal out"=w52:waveform(dbl))  [unwired: 5 in, 1 out]
  n78 = call-poly <vilib>:"Append Waveforms.vi"("waveform B"=w52, "waveform A"=w47) -> ("waveform out"=w45:waveform(dbl))  [unwired: 8 in, 1 out]
  n79 = call "XYWaveform.vi"("XYWaveformIN"=w4) -> ("XYWaveformOut"=w42:waveform(dbl))  [unwired: 10 in]
  n80 = call "XYWaveform.vi"("XYWaveformIN"=w3) -> ("XYWaveformOut"=w41:waveform(dbl))  [unwired: 10 in]
  n81 = call "XYWaveform.vi"("XYWaveformIN"=w29) -> ("XYWaveformOut"=w38:waveform(dbl))  [unwired: 10 in]
  n82 = Bundle By Name(cluster="SetupInfo_IN", "AnalogWaveform.Bi-lateral Galvo XY stand waveform"=w75, "AnalogWaveform.Bi-lateral Galvo XY OG waveform"=w136, "AnalogWaveform.Frontal Galvo XY OG waveform"=w132, "AnalogWaveform.Frontal Galvo XY stand waveform"=w129, "AnalogWaveform.Bi-lateral Galvo Z stand waveform"=w4, "AnalogWaveform.Frontal Galvo Z stand waveform"=w3, "AnalogWaveform.Detection objective stand waveform"=w29, "AnalogWaveform.sCMOS stand waveform"=w40, "AnalogWaveform.sCMOS blank waveform"=w123, "AnalogWaveform.PFI 0 clock stand waveform"=w122, "AnalogWaveform.AOM stand waveform"=w36, "DigitalWaveform.Plane Indexing"=w68, "AnalogWaveform.Bi-lateral Galvo Z OG waveform"=w70, "AnalogWaveform.Frontal Galvo Z OG waveform"=w69, "AnalogWaveform.Detection objective OG waveform"=w57, "AnalogWaveform.sCMOS OG waveform"=w45, "DigitalWaveform.Plane indexing P0.5 OG"=w79, "AnalogWaveform.PFI 0 clock OG wavee"=w78, "AnalogWaveform.AOM OG waveform"=w77, "AnalogWaveform.Bi-lateral Galvo Z XY"=w42, "AnalogWaveform.Frontal Galvo Z XY"=w41, "AnalogWaveform.sCMOS Trigger XY"=w39, "AnalogWaveform.Detection objective XY"=w38, "AnalogWaveform.AOM XY"=w37) -> (→"SetupInfo_OUT":T1)
  "error out" <- "error in (no error)"
